vi "Engine.vi"(8 "error in (no error)":errorcluster, 11 "ModbusSp in":refnum<class "ModbusSp.lvclass">) -> (0 "error out":errorcluster, 3 "ModbusSp out":refnum<class "ModbusSp.lvclass">)   [LabVIEW 2019, in "ModbusSp.lvclass"]
uses:
  ModbusSp.lvclass
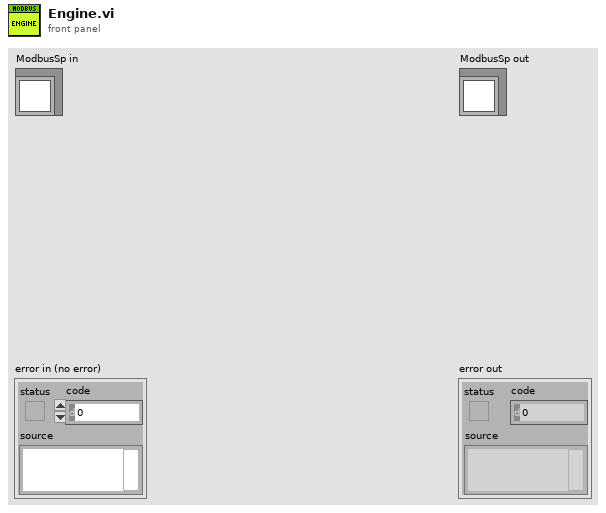
[diagram p1: front panel]
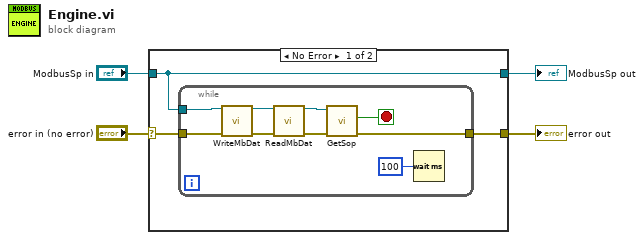
[diagram p0: block diagram]
diagram:
  n1 = case shown="No Error" "error in (no error)" {
    selector: "error in (no error)" -> [w7 w18]
    tunnel: [w6 w18] -> w3
    tunnel: [w5 w17] -> w1
    tunnel: "ModbusSp in" -> [w5 w17]
    frame No Error {
      n2 = while {
        tunnel: w5 -> [w16]
        tunnel: w7 -> [w15]
        tunnel: [w8] -> w6
        stop <- w9 stop-if-true
        n3 = call "WriteMbDat.vi"("ModbusSp in"=w16, "error in (no error)"=w15) -> ("ModbusSp out"=w14:refnum<class "ModbusSp.lvclass">, "error out"=w13:errorcluster)  [unwired: 12 in]
        n4 = call "ReadMbDat.vi"("ModbusSp in"=w14, "error in (no error)"=w13) -> ("ModbusSp out"=w11:refnum<class "ModbusSp.lvclass">, "error out"=w10:errorcluster)  [unwired: 12 in]
        n5 = call "GetSop.vi"("error in (no error)"=w10, "ModbusSp in"=w11) -> ("error out"=w8:errorcluster, "value"=w9:bool)  [unwired: 7 in, 1 out]
        n6 = Wait (ms)(milliseconds to wait=u32 100) -> ()  [unwired: 1 out]
      }
    }
    frame Error {
    }
  }
  "error out" <- w3
  "ModbusSp out" <- w1
